vi "Step Core.vi"(8 "error in (no error)":errorcluster, 11 "NF in":refnum<class "NF.lvclass">) -> (0 "error out":errorcluster, 3 "NF out":refnum<class "NF.lvclass">)   [LabVIEW 2018, in "NF.lvlib" / "NF.lvclass"]
uses:
  NF.lvclass
  Plugins/Measurement Interface.lvlibp/Measurement Interface.lvclass
  C:/Sequence Automation/Plugins/Measurement Interface.lvlibp/Measurement Interface.lvclass
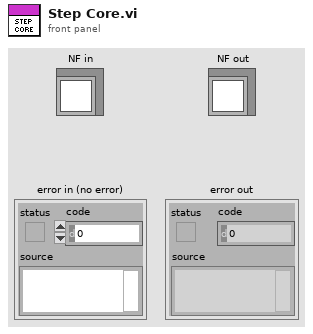
[diagram p1: front panel]
types:
  T1 = typedef "TestStand API Tools (TSAT).lvlibp/TSAT Evaluation Actions.lvlib/TSAT Evaluation.ctl" = cluster{"Test Name":string, "Pin":string, "Units":string, "SI Scaling":T2, "Test Number":i32, "Published Data Id":string, "Low Limit":dbl, "High Limit":dbl, "Export Data Location":string, "Software Bin":i64, "Evaluation Type":T3, "Test Data Source":string}
  T2 = typedef "TestStand API Tools (TSAT).lvlibp/TSAT Evaluation Actions.lvlib/TSAT Eval SI Unit Scaling.ctl" = i16
  T3 = typedef "TestStand API Tools (TSAT).lvlibp/TSAT Evaluation Actions.lvlib/TSAT Evaluation Type.ctl" = enum16{"Numeric Limit", "Pass/Fail", "None"}
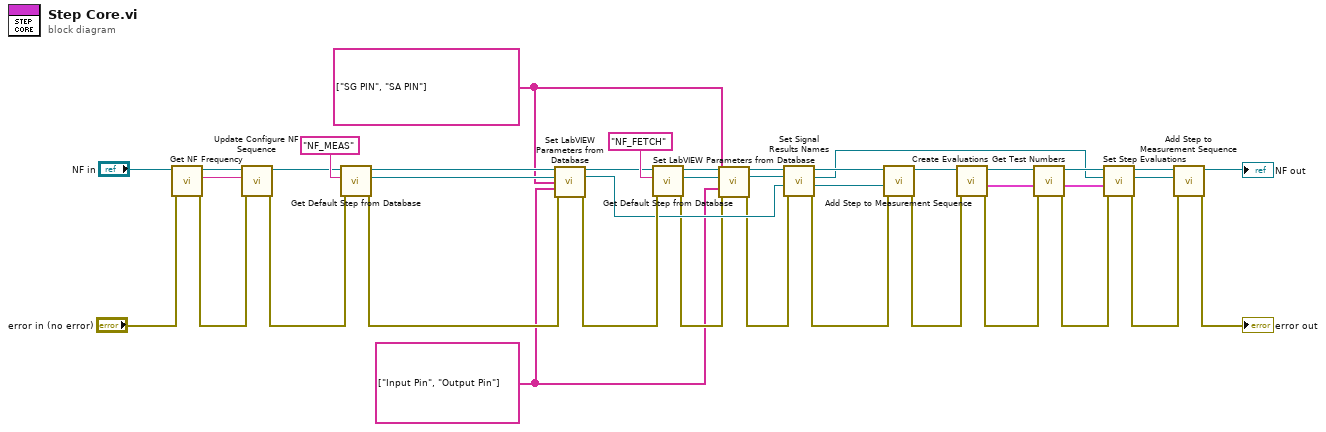
[diagram p0: block diagram]
diagram:
  w15 = string[] ["Input Pin", "Output Pin"] ("LabVIEW Parameter Mapping")
  w16 = string[] ["SG PIN", "SA PIN"] ("Dictionary Keys")
  n1 = call-dynamic "Get NF Frequency.vi"("error in (no error)"="error in (no error)", "NF in"="NF in") -> ("error out"=w33:errorcluster, "NF frequency"=w32:string, "NF out"=w35:refnum<class "NF.lvclass">)  [unwired: 7 in]
  n2 = call-dynamic "Update Configure NF Sequence.vi"("error in (no error)"=w33, "NF Freq (Hz)"=w32, "NF in"=w35) -> ("error out"=w38:errorcluster, "NF out"=w39:refnum<class "NF.lvclass">)  [unwired: 7 in]
  n3 = call "Get Default Step from Database.vi"("error in (no error)"=w38, "Default Step"="NF_MEAS", "Measurement Interface in"=w39) -> ("error out"=w30:errorcluster, "Cloned Step"=w29:refnum<k7>, "Measurement Interface out"=w31:refnum<class "NF.lvclass">)  [unwired: 6 in]
  n4 = call "Set LabVIEW Parameters from Database.vi"("Measurement Interface in"=w31, "Step In"=w29, "Dictionary Keys"=w16, "LabVIEW Parameter Mapping"=w15, "error in (no error)"=w30) -> ("Measurement Interface out"=w27:refnum<class "NF.lvclass">, "Step Out"=w26:refnum<k7>, "error out"=w28:errorcluster)  [unwired: 8 in]
  n5 = call "Get Default Step from Database.vi"("error in (no error)"=w28, "Default Step"="NF_FETCH", "Measurement Interface in"=w27) -> ("error out"=w20:errorcluster, "Cloned Step"=w18:refnum<k7>, "Measurement Interface out"=w22:refnum<class "NF.lvclass">)  [unwired: 6 in]
  n6 = call "Set LabVIEW Parameters from Database.vi"("Measurement Interface in"=w22, "Step In"=w18, "Dictionary Keys"=w16, "LabVIEW Parameter Mapping"=w15, "error in (no error)"=w20) -> ("Measurement Interface out"=w21:refnum<class "NF.lvclass">, "Step Out"=w17:refnum<k7>, "error out"=w19:errorcluster)  [unwired: 8 in]
  n7 = call-dynamic "Set Signal Results Names.vi"("error in (no error)"=w19, "Meas Step Ref"=w26, "Fetch Step Ref"=w17, "NF in"=w21) -> ("error out"=w24:errorcluster, "Meas Step Ref"=w23:refnum<k7>, "Fetch Step Ref"=w5:refnum<k7>, "NF out"=w25:refnum<class "NF.lvclass">)  [unwired: 4 in]
  n8 = call "Add Step to Measurement Sequence.vi"("error in (no error)"=w24, "Step to Add"=w23, "Measurement Interface in"=w25) -> ("error out"=w8:errorcluster, "Measurement Interface out"=w10:refnum<class "NF.lvclass">)  [unwired: 7 in]
  n9 = call-dynamic "Create Evaluations.vi"("error in (no error)"=w8, "NF in"=w10) -> ("error out"=w13:errorcluster, "Evaluations Out"=w3:T1[], "NF out"=w14:refnum<class "NF.lvclass">)  [unwired: 7 in]
  n10 = call-dynamic "Get Test Numbers.vi"("error in (no error)"=w13, "NF Evaluations In"=w3, "NF in"=w14) -> ("error out"=w11:errorcluster, "NF Evaluations Out"=w2:T1[], "NF out"=w12:refnum<class "NF.lvclass">)  [unwired: 6 in]
  n11 = call-dynamic "Set Step Evaluations.vi"("error in (no error)"=w11, "Evaluation Data"=w2, "Step In"=w5, "NF in"=w12) -> ("error out"=w7:errorcluster, "Step Out"=w4:refnum<k7>, "NF out"=w9:refnum<class "NF.lvclass">)  [unwired: 5 in]
  n12 = call "Add Step to Measurement Sequence.vi"("error in (no error)"=w7, "Step to Add"=w4, "Measurement Interface in"=w9) -> ("error out"=→"error out":errorcluster, "Measurement Interface out"=→"NF out":refnum<class "NF.lvclass">)  [unwired: 7 in]
